vi "SR430_bins_per_record_2_bins.vi"(2 "binsPerRecord":i32, 5 "error in (no error)":errorcluster) -> (16 "bins":i32, 17 "In Range?":bool, 19 "error out":errorcluster)   [LabVIEW 2009, in "SR430Driver.lvlib"]
doc: "converts number of bins per record in the format as used by the unit into a user friendly format.VI Tree for the SR430 Multi-Channel Scaler from Staford Research Systems.\n\nHistory: 24-APR-2002, Dietrich Beck\n\nCopyright (C)\nGesellschaft für Schwerionenforschung, GSI\nPlanckstr. 1\n64291 Darmstadt\nGermany\n\nContact: D.Beck@gsi.de \n\nThis program is free software; you can redistribute it and/or modify it under the terms of the \nGNU General Public License as published by the Free Software Foundation; either version 2 of the license, or (at your option) any later version.\n\nThis program is distributed in the hope that it will be useful, but WITHOUT ANY WARRANTY; without even the implied warranty of MERCHANTABILITY or FITNESS FOR A PARTICULAR PURPOSE. See the GNU General License for more details (http://www.gnu.org).\n\nGesellschaft für Schwerionenforschung, GSI\nPlanckstr. 1, 64291 Darmstadt, Germany\nFor all questions and ideas contact: M.Richter@gsi.de, K.Poppensieker, H.Brand@gsi.de or D.Beck@gsi.de.\nLast update: 11-APR-2002"
uses:
  SR430Driver.lvlib
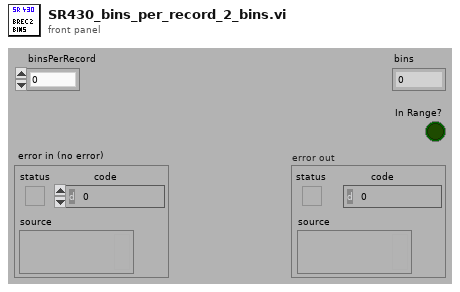
[diagram p1: front panel]
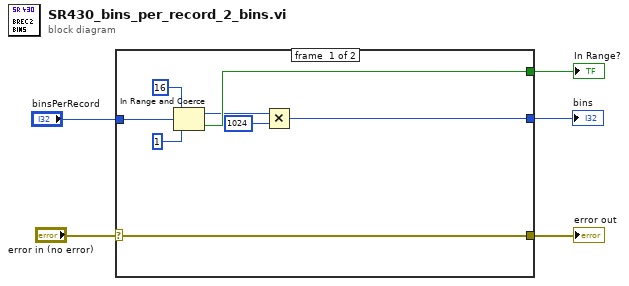
[diagram p0: block diagram]
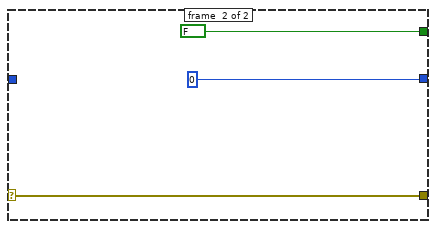
[diagram p2: hidden frame]
diagram:
  n1 = case shown="No Error" "error in (no error)" {
    selector: "error in (no error)" -> [w13 w16]
    tunnel: [w13 w16] -> w4
    tunnel: "binsPerRecord" -> [w12 _]
    tunnel: [w9 FALSE] -> w3
    tunnel: [w6 0] -> w1
    frame #0 {
      n2 = In Range and Coerce(upper limit=16, x=w12, lower limit=1) -> (coerced(x)=w8:i32, In Range?=w9:bool)
      n3 = Multiply(x=w8, y=1024) -> (x*y=w6:i32)
    }
    frame #1 {
    }
  }
  "error out" <- w4
  "bins" <- w1
  "In Range?" <- w3
